vi "init connection.vi"(8 "error in (no error)":errorcluster, 9 "server port":i32, 10 "server ip":string, 11 "tcp server connection in":refnum<class "tcp server connection.lvclass">) -> (0 "error out":errorcluster, 3 "tcp server connection out":refnum<class "tcp server connection.lvclass">)   [LabVIEW 2014, in "tcp server connection.lvclass"]
uses:
  tcp server connection.lvclass
  typedefs/connection type.ctl
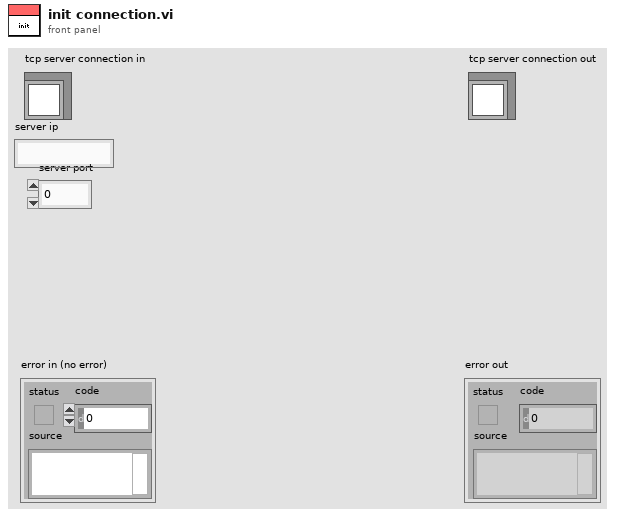
[diagram p1: front panel]
types:
  T1 = typedef "connection type.ctl" = enum16{"client", "server"}
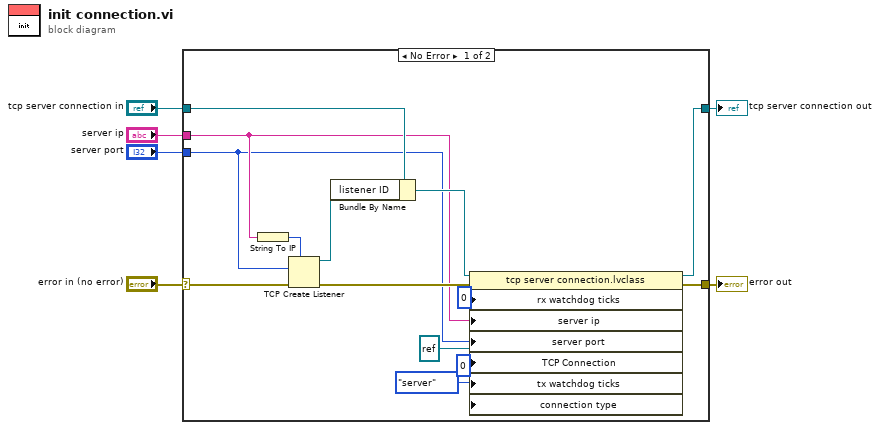
[diagram p0: block diagram]
diagram:
  n1 = case shown="No Error" "error in (no error)" {
    selector: "error in (no error)" -> [w19 w22]
    tunnel: [w13 w22] -> w5
    tunnel: [w16 w21] -> w3
    tunnel: "tcp server connection in" -> [w17 w21]
    tunnel: "server ip" -> [w9 _]
    tunnel: "server port" -> [w8 _]
    frame No Error {
      n2 = String To IP(1:w9) -> (0:w20:u32)
      n3 = TCP Create Listener(7:w20, 8:w19, 10:w8) -> (0:w14:errorcluster, 3:w18:refnum<k5>)  [unwired: 2 in, 1 out]
      n4 = Bundle By Name(cluster=w17, "listener ID"=w18) -> (w15:refnum<class "tcp server connection.lvclass">)
      n5 = property class="tcp server connection.lvclass"(reference=w15, error in=w14, "rx watchdog ticks"=u32 0 ("tx watchdog ticks"), "server ip"=w9, "server port"=w8, "TCP Connection"=refnum<k5> refnum, "tx watchdog ticks"=u32 0, "connection type"=connection_type."server") -> (reference out=w16:refnum<class "tcp server connection.lvclass">, error out=w13:errorcluster)
    }
    frame Error {
    }
  }
  "error out" <- w5
  "tcp server connection out" <- w3
